vi "AdaptedForYb.vi"() -> ()   [LabVIEW 2017, in "GP22_TDC_Arduinoed.lvlib"]
uses:
  GP22_TDC_Arduinoed.lvlib
  <vilib>/express/express analysis/Spectral/Block/exnSpectralBlock spectral measurements peak poly.vi
  <vilib>/express/express analysis/Spectral/Block/exnSpectralBlock spectral measurements peak DDT.vi
  <vilib>/express/express analysis/Spectral/XNode/ExpressSpectralMeasurementsBlockNode.xnode
  <vilib>/Analysis/NI_AALBase.lvlib
  <vilib>/Analysis/baseanly.llb/Mean (DBL).vi
panel:
  out "Num.readings":i32
  in  "Time in ms (30000)":u32=5000
  in  "VISA resource name":refnum<visa-resource-name>="COM6"
  out "Binned":dbl[](graph) caption="best fit"
  out "Phase history":dbl(graph)=1.2687322673619421
  out "mean":dbl=5.726 format="%0.2f"
  out "mod depth":dbl=0.18964378272179214 format="%#_3g"
  out "Peak phase":dbl=1.2687322673619421
  out "Peak history":dbl(graph)=0.18964378272179214
  out "Peak height":dbl=1.0859002998649818 format="%#_4g"
  out "FFT":dbl[](graph) caption="best fit"
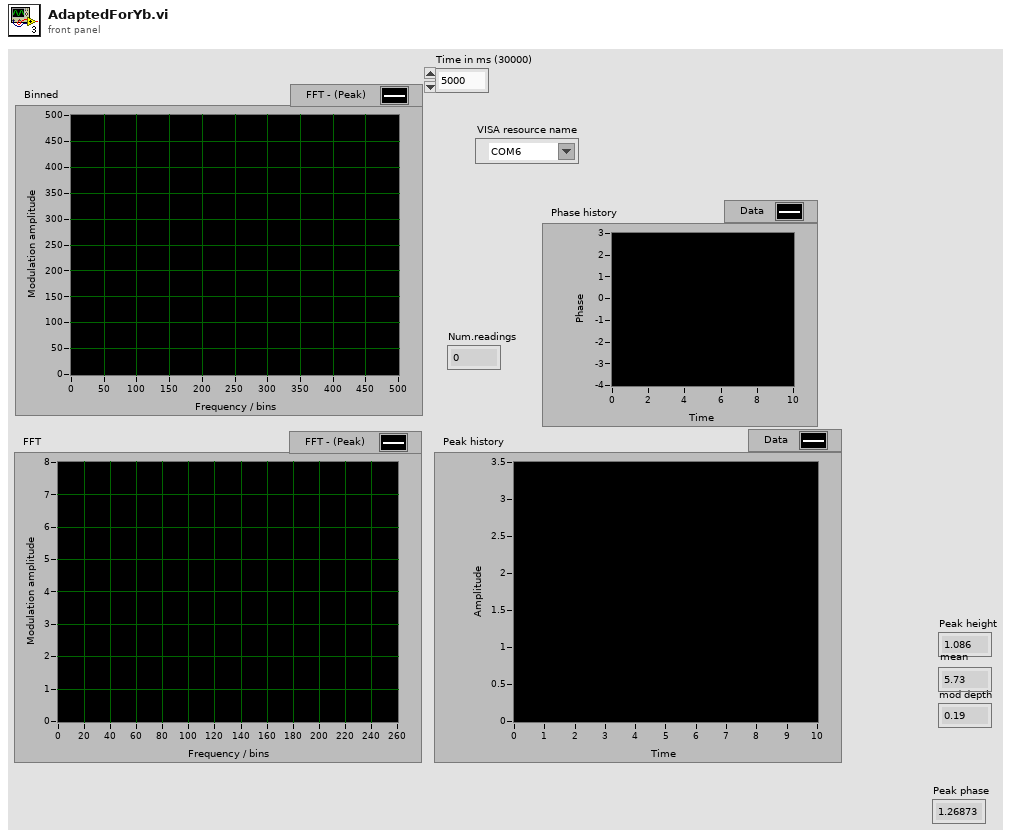
[diagram p1: front panel]
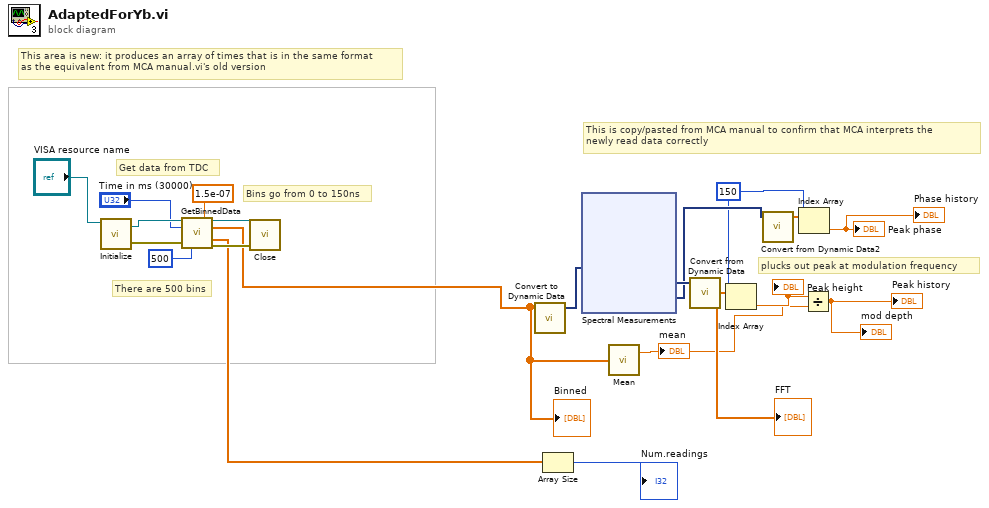
[diagram p0: block diagram]
diagram:
  w14 = 150
  # "This is copy/pasted from MCA manual to confirm that MCA interprets the \nnewly read data correctly"
  # "This area is new: it produces an array of times that is in the same format \nas the equivalent from MCA manual.vi's old version"
  # "There are 500 bins"
  # "Bins go from 0 to 150ns"
  # "Get data from TDC"
  # "plucks out peak at modulation frequency"
  n1 = call "Initialize.vi"("VISA resource name"="VISA resource name") -> ("error out"=w7:errorcluster, "VISA resource name out"=w10:refnum<visa-resource-name>)  [unwired: 5 in]
  n2 = call "GetBinnedData.vi"("VISA resource name"=w10, "Maximum Value"=1.5e-07, "Time in ms (30000)"="Time in ms (30000)", "error in"=w7, "# bins"=500) -> ("VISA resource name out"=w9:refnum<visa-resource-name>, "Binned time"=w3:dbl[], "Unbinned times / s"=w1:dbl[], "error out"=w8:errorcluster)  [unwired: 7 in]
  "Binned" <- w3
  n3 = call "Close.vi"("error in (no error)"=w8, "VISA resource name"=w9) -> ()  [unwired: 9 in, 1 out]
  n4 = call "Convert to Dynamic Data"("Array"=w3) -> ("Dynamic Data Type"=w21:dynamicdata)  [unwired: 3 in]
  n5 = Array Size(array=w1) -> (size(s)=→"Num.readings":i32)
  n6 = xnode "Spectral Measurements"("Signals"=w21) -> ("FFT - (Peak)"=w20:dynamicdata, "Phase"=w17:dynamicdata)  [unwired: 1 in, 1 out]
  n7 = call-poly <vilib>:"Mean.vi"("X"=w3) -> ("mean"=w15:dbl)  [unwired: 1 out]
  "mean" <- w15
  n8 = call "Convert from Dynamic Data"("Dynamic Data Type"=w20) -> ("Array"=w19:dbl[])  [unwired: 3 in]
  "FFT" <- w19
  n9 = Index Array(array=w19, index=w14) -> (element=w18:dbl)
  "Peak height" <- w18
  n10 = call "Convert from Dynamic Data2"("Dynamic Data Type"=w17) -> ("Array"=w16:dbl[])  [unwired: 3 in]
  n11 = Index Array(array=w16, index=w14) -> (element=→"Peak phase" →"Phase history":dbl)
  n12 = Divide(x=w18, y=w15) -> (x/y=→"Peak history" →"mod depth":dbl)
